vi "AddData.vi"() -> (2 "?":bool, 3 "ProgramData 2":T1={"Numer Produktu"="abc", "Nazwa Produktu"="dd", "Wytwórca"="ss"})   [LabVIEW 2018]
uses:
  ProductsCluster.ctl
panel:
  in  "ProgramData":T1
  in  "Cancel Button":bool
  in  "OK Button":bool
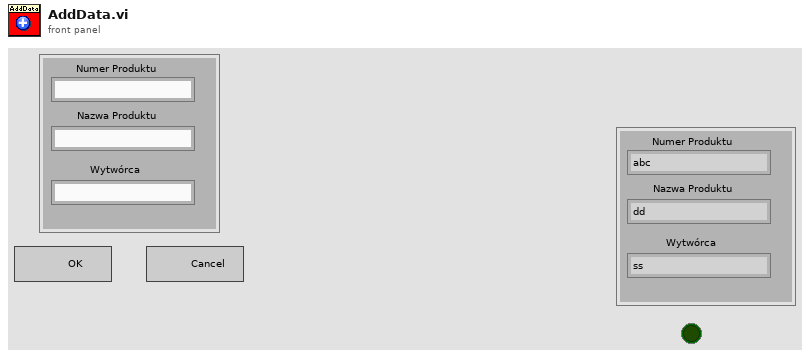
[diagram p1: front panel]
types:
  T1 = typedef "ProductsCluster.ctl" = cluster{"Numer Produktu":string, "Nazwa Produktu":string, "Wytwórca":string}
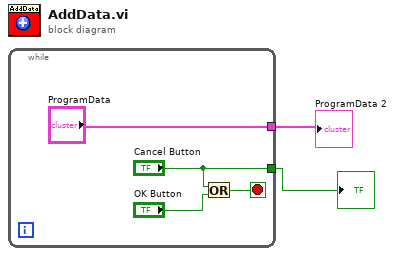
[diagram p0: block diagram]
diagram:
  n1 = while {
    tunnel: ["ProgramData"] -> w1
    tunnel: ["Cancel Button"] -> w2
    stop <- w5 stop-if-true
    n2 = Or(x="Cancel Button", y="OK Button") -> (x .or. y?=w5:bool)
  }
  "?" <- w2
  "ProgramData 2" <- w1
